vi "Servo Controller.vi"(6 "Enum":enum16{"Door", "Wiper"}(ring)=enum."Wiper", 8 "Wiper Flag":bool, 9 "Servo Period":dbl, 10 "Duty min":dbl, 11 "Door":bool) -> (0 "Wiper Flag Shift Reg":bool, 2 "Shift Reg":dbl, 3 "Door Duty":dbl)   [LabVIEW 2015]
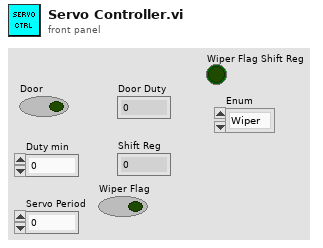
[diagram p1: front panel]
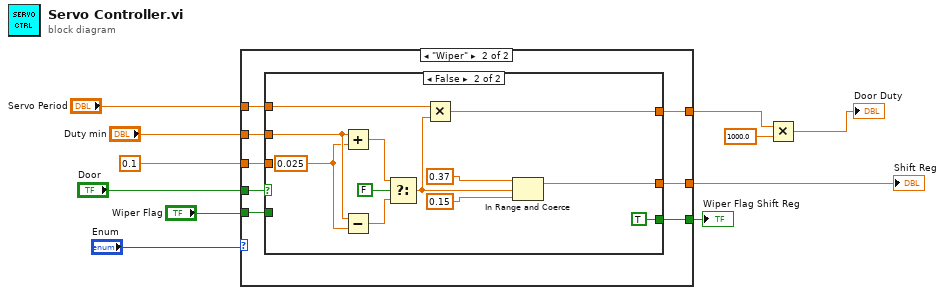
[diagram p0: block diagram]
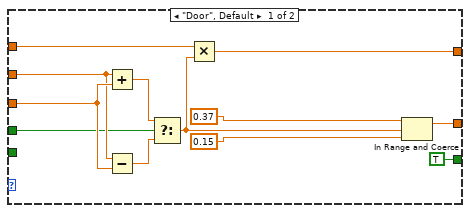
[diagram p2: hidden frame]
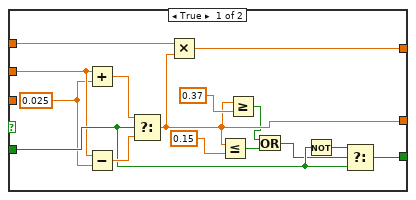
[diagram p3: hidden frame]
diagram:
  n1 = case shown="\"Wiper\"" "Enum" {
    tunnel: 0.1 ("y") -> [w23 w30]
    tunnel: "Duty min" -> [w22 w25]
    tunnel: [w21 w27] -> w3
    tunnel: "Servo Period" -> [w19 w26]
    tunnel: [w18 w28] -> w8
    tunnel: "Door" -> [w13 w31]
    tunnel: "Wiper Flag" -> [_ w29]
    tunnel: [TRUE ("Wiper Flag") w24] -> w4
    frame "Door", Default {
      n2 = Add(x=w22, y=w23) -> (x+y=w14:dbl)
      n3 = Subtract(x=w22, y=w23) -> (x-y=w15:dbl)
      n4 = Select(t=w14, s=w13, f=w15) -> (s? t:f=w20:dbl)
      n5 = Multiply(x=w19, y=w20) -> (x*y=w21:dbl)
      n6 = In Range and Coerce(upper limit=0.37, x=w20, lower limit=0.15 ("upper limit")) -> (coerced(x)=w18:dbl)  [unwired: 1 out]
    }
    frame "Wiper" {
      n7 = case shown="False" w31 {
        tunnel: w30 -> [_ _]
        tunnel: w29 -> [w41 _]
        tunnel: [w37 w53] -> w28
        tunnel: [w44 w52] -> w27
        tunnel: w26 -> [w43 w51]
        tunnel: w25 -> [w39 w48]
        tunnel: [w42 TRUE ("Wiper Flag")] -> w24
        frame True {
          w32 = 0.025 ("y")
          n8 = Add(x=w39, y=w32) -> (x+y=w45:dbl)
          n9 = Subtract(x=w39, y=w32) -> (x-y=w46:dbl)
          n10 = Select(t=w45, s=w41, f=w46) -> (s? t:f=w37:dbl)
          n11 = Multiply(x=w43, y=w37) -> (x*y=w44:dbl)
          n12 = Less Or Equal?(x=w37, y=0.15 ("upper limit")) -> (x <= y?=w35:bool)
          n13 = Greater Or Equal?(x=w37, y=0.37 ("upper limit")) -> (x >= y?=w34:bool)
          n14 = Or(x=w34, y=w35) -> (x .or. y?=w33:bool)
          n15 = Not(x=w41) -> (.not. x?=w40:bool)
          n16 = Select(t=w40, s=w33, f=w41) -> (s? t:f=w42:bool)
        }
        frame False {
          w47 = 0.025 ("y")
          n17 = Add(x=w48, y=w47) -> (x+y=w54:dbl)
          n18 = Subtract(x=w48, y=w47) -> (x-y=w55:dbl)
          n19 = Select(t=w54, s=FALSE, f=w55) -> (s? t:f=w58:dbl)
          n20 = Multiply(x=w51, y=w58) -> (x*y=w52:dbl)
          n21 = In Range and Coerce(upper limit=0.37, x=w58, lower limit=0.15 ("upper limit")) -> (coerced(x)=w53:dbl)  [unwired: 1 out]
        }
      }
    }
  }
  "Shift Reg" <- w8
  "Wiper Flag Shift Reg" <- w4
  n22 = Multiply(x=w3, y=1000.0) -> (x*y=→"Door Duty":dbl)
